vi "Q8381 Wave Data Change to Array.vi"(1 "Receive Data":string, 2 "Data Number":u16) -> (0 "Data Array":dbl[](array[numeric]) format="%.5e")   [LabVIEW 2017]
panel:
  in  "Data Change offset":u16
  # "Wave Data Change to Array"
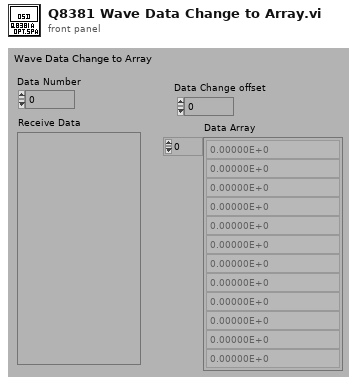
[diagram p1: front panel]
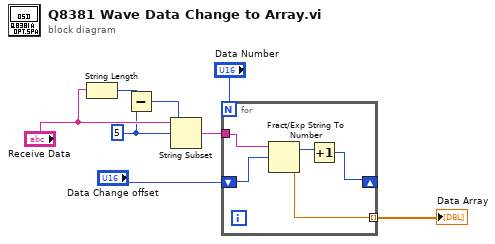
[diagram p0: block diagram]
diagram:
  w6 = 5
  n1 = String Length(string="Receive Data") -> (length=w7:i32)
  n2 = Subtract(x=w7, y=w6) -> (x-y=w5:i32)
  n3 = String Subset(string="Receive Data", offset (0)=w6, length (rest)=w5) -> (substring=w3:string)
  n4 = for {
    N: "Data Number" -> [_]
    shift-right: [w9] -> _
    shift-left: "Data Change offset" -> [w10]
    tunnel: w3 -> [w12]
    tunnel: [w11] -> w2 mode=indexing
    n5 = Fract/Exp String To Number(string=w12, offset=w10) -> (offset past number=w13:i32, number=w11:dbl)  [unwired: 2 in]
    n6 = Increment(x=w13) -> (x+1=w9:i32)
  }
  "Data Array" <- w2
